vi "Untitled 6 (SubVI).vi"(0 "x(t-1)":dbl[](array[numeric]), 1 "x(t)":dbl[](array[numeric]), 2 "x(t-2)":dbl[](array[numeric]), 3 "y(t-1)":dbl[](array[numeric]), 4 "smooth window size":dbl, 5 "y(t-2)":dbl[](array[numeric]), 8 "RC y(t-1)":dbl[](array[numeric])) -> (6 "smoothed data":dbl[](array[numeric]))   [LabVIEW 2009]
panel:
  in  "method":i32=1
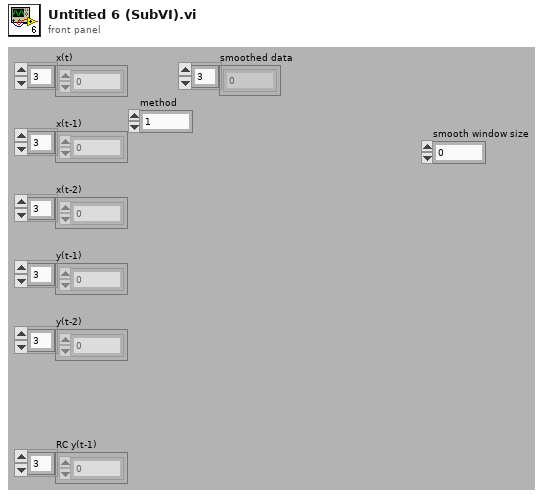
[diagram p1: front panel]
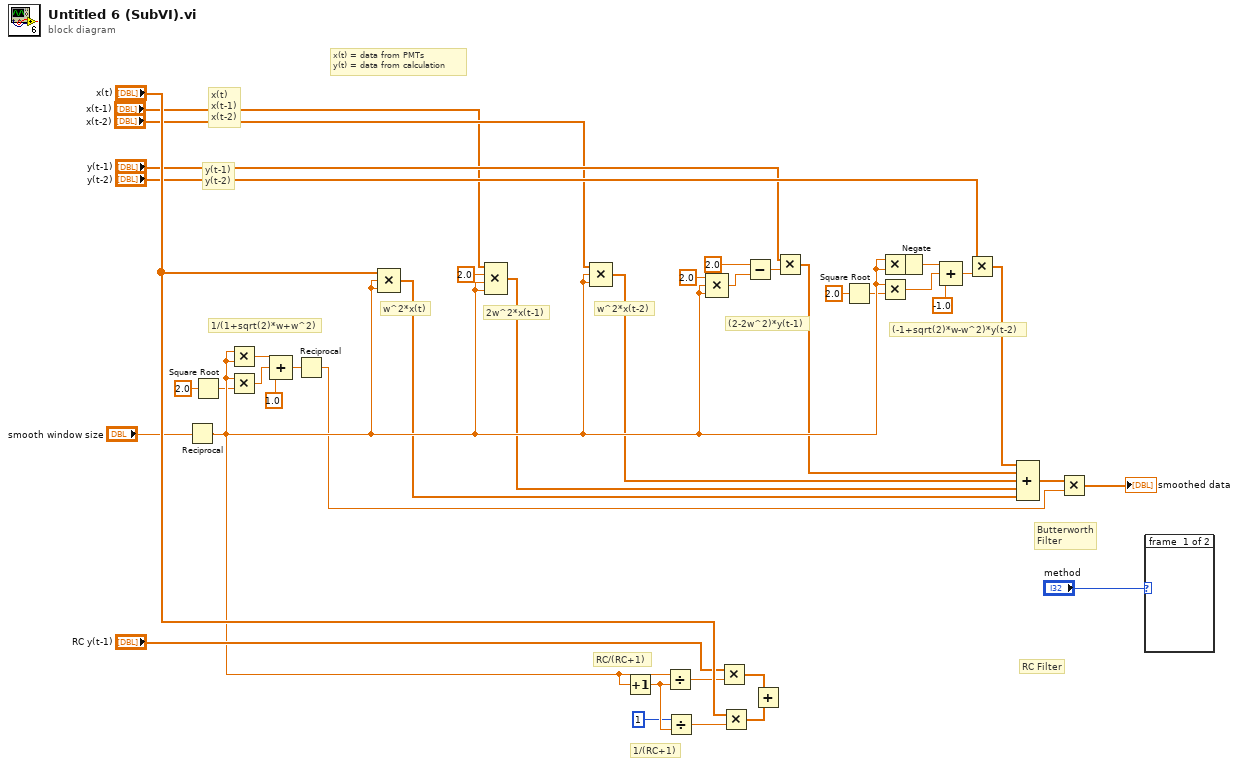
[diagram p0: block diagram]
diagram:
  # "x(t) = data from PMTs\ny(t) = data from calculation"
  # "y(t-1)\ny(t-2)"
  # "x(t)\nx(t-1)\nx(t-2)"
  # "Butterworth\nFilter"
  # "RC Filter"
  # "1/(RC+1)"
  # "RC/(RC+1)"
  # "(2-2w^2)*y(t-1)"
  # "(-1+sqrt(2)*w-w^2)*y(t-2)"
  # "w^2*x(t-2)"
  # "2w^2*x(t-1)"
  # "w^2*x(t)"
  # "1/(1+sqrt(2)*w+w^2)"
  n1 = Reciprocal(x="smooth window size") -> (1/x=w40:dbl)
  n2 = Square Root(x=2.0 ("y")) -> (sqrt(x)=w9:dbl)
  n3 = Multiply(x=w40, y=w40) -> (x*y=w3:dbl)
  n4 = Multiply(x=w40, y=w9) -> (x*y=w4:dbl)
  n5 = Compound Arithmetic op=ADD(w3, w4, 1.0 ("y")) -> (w6:dbl)
  n6 = Reciprocal(x=w6) -> (1/x=w27:dbl)
  n7 = Compound Arithmetic op=MULTIPLY("x(t)", w40, w40) -> (w25:dbl[])
  n8 = Compound Arithmetic op=MULTIPLY("x(t-1)", 2.0 ("y"), w40, w40) -> (w24:dbl[])
  n9 = Compound Arithmetic op=MULTIPLY("x(t-2)", w40, w40) -> (w23:dbl[])
  n10 = Increment(x=w40) -> (x+1=w38:dbl)
  n11 = Divide(x=w40, y=w38) -> (x/y=w37:dbl)
  n12 = Divide(x=1 ("smooth size"), y=w38) -> (x/y=w39:dbl)
  n13 = Compound Arithmetic op=MULTIPLY(2.0 ("value"), w40, w40) -> (w18:dbl)
  n14 = Multiply(x="RC y(t-1)", y=w37) -> (x*y=w35:dbl[])
  n15 = Multiply(x="x(t)", y=w39) -> (x*y=w36:dbl[])
  n16 = Subtract(x=2.0 ("value"), y=w18) -> (x-y=w20:dbl)
  n17 = Add(x=w35, y=w36) -> (x+y=w33:dbl[])
  n18 = Multiply(x="y(t-1)", y=w20) -> (x*y=w22:dbl[])
  n19 = Square Root(x=2.0 ("y")) -> (sqrt(x)=w10:dbl)
  n20 = Multiply(x=w40, y=w40) -> (x*y=w13:dbl)
  n21 = Multiply(x=w40, y=w10) -> (x*y=w12:dbl)
  n22 = Negate(x=w13) -> (-x=w15:dbl)
  n23 = Compound Arithmetic op=ADD(w15, w12, -1.0 ("y")) -> (w16:dbl)
  n24 = Multiply(x="y(t-2)", y=w16) -> (x*y=w21:dbl[])
  n25 = Compound Arithmetic op=ADD(w21, w22, w23, w24, w25) -> (w26:dbl[])
  n26 = Multiply(x=w26, y=w27) -> (x*y=→"smoothed data":dbl[])
  n27 = case shown="1" "method" {
    frame #0 {
    }
    frame #1 {
    }
  }
